vi "__file_name.vi"(8 "comment2":string="m", 9 "種類":u16(ring)=12 items=["LOopt", "LO sweep", "I-V", "I-V NOLO", "I-V Trx", "SP", "YIG", "SBR", "allan", "Gain comp", "Cross Talk", "-----", "A_YIG", "A_SBR", "AL_allan", "AL_fft", "AL_temp", "AL_data", "shapiro", "JC", "htr", "A_SP"], 10 "Control":T2={"GPIB_ATT"="28", "6501Dev#"=1, "GPIB_SP"="18", "GPIB_PM"="13", "GPIB_DSA"="11", "GPIB_DMM (TPD)"="23", "GPIB_MPI"="COM5", "mortor設定"=[{"Axis"=0, "ID"=0, "HIspeed"=200.0, "LOspeed"=100.0, "ACCEL(ms)"=100.0, "Sratio"=50.0, "フリーラン\n"=FALSE, "文字列"="DSB HOT/COLD"}, {"Axis"=1, "ID"=0, "HIspeed"=4.0, "LOspeed"=4.0, "ACCEL(ms)"=100.0, "Sratio"=50.0, "フリーラン\n"=TRUE, "文字列"="SubMM Att"}, {"Axis"=0, "ID"=0, "HIspeed"=200.0, "LOspeed"=100.0, "ACCEL(ms)"=100.0, "Sratio"=50.0, "フリーラン\n"=FALSE, "文字列"="MPI Port1"}, {"Axis"=1, "ID"=0, "HIspeed"=200.0, "LOspeed"=100.0, "ACCEL(ms)"=100.0, "Sratio"=50.0, "フリーラン\n"=FALSE, "文字列"="MPI Port2"}, {"Axis"=1, "ID"=0, "HIspeed"=200.0, "LOspeed"=100.0, "ACCEL(ms)"=100.0, "Sratio"=50.0, "フリーラン\n"=TRUE, "文字列"="gainComp"}], "DATAパス"=path "L:/cartridge/assembly/SN03/03-13/110628_WCADSB_P0", "DBパス "=path "Z:/band10/Labview_ALMA/MIX95/test", "comment"="110628_WCADSB_P0", "ColdCarts"="003601", "Th"=299.0, "Tc"=83.0, "Set_SIS_volt"=2.1, "Offset"=0.0, "control"=0, "FreqLO"=799.0, "Set_Mag_Cur"=8.86861313868613, "MPI offset(mm)"=23.166, "HOT/COLD"=0} {"HOT/COLD" items=["DSB", "SBR (Cart.)", "GainComp", "SBR (MIX)"]; "control" items=["CLOSE LOOP", "OPEN LOOP", "Not Control"]}, 11 "Bias_LO_equip":T1={"Node address"=19, "CAN Interface"="CAN0", "Cartridge band"=10, "Slave Node in"={"Address"=19, "Serial Number"=[16, -88, -112, 75, 1, 8, 0, 24]}, "ObjHandle out"=93257792, "POL"=0, "sb"=1, "GPIB_SM (SIS S,V)"="24", "GPIB_DMM (SIS I)"="22", "GPIB_SM (MAG I) "="25", "GPIB_SG(LO)"="19", "GPIB_PW (PAMP) "="6", "GPIB_TMP1(8ch)"="12", "GPIB_TMP2(2ch)  "="13", "WCA_avg"=10, "Rsen"=10.0, "BiasModule"=1, "LOModule "=2, "WCA_LO_FREQ_SET"={"YTO Low freq. [GHz]"=14.66, "YTO High freq. [GHz]"=17.5, "Kvco"=1, "Lock Pol."=0, "SET LO FREQ"=97.111115, "Multiplier"=6.0, "YTO (HEX)"=2196, "YTO ( FREQ)"=16.18299, "NULL PLL INTEGRATOR"=FALSE}, "Res for"=0} {"Res for" items=["none", "series res", "parallel res"]; "WCA_LO_FREQ_SET"."YTO ( FREQ)" min=25 max=150 step=0.0001 format="%.3f"; "WCA_LO_FREQ_SET"."Multiplier" min=3 max=6 step=3; "WCA_LO_FREQ_SET"."SET LO FREQ" min=25 max=150 step=0.0001 format="%.3f"; "WCA_LO_FREQ_SET"."Lock Pol." items=["Lower", "Upper"]; "WCA_LO_FREQ_SET"."Kvco" items=["7.5MHz/V", "15MHz/V"]; "WCA_LO_FREQ_SET"."YTO High freq. [GHz]" format="%.3f"; "WCA_LO_FREQ_SET"."YTO Low freq. [GHz]" format="%.3f"; "LOModule" items=["Manual Gunn+PAMP"=0, "PLL GUNN+PAMP"=5, "B10Lab LO"=1, "WCA LO"=2, ""=3, "YIG発信器"=4, "none"=99]; "BiasModule" items=["B10Lab Bias"=0, "WCA BiasModule"=1, "none"=99]; "Slave Node in"."Serial Number" format="%.0x"; "Slave Node in"."Address" format="%.0x"; "Cartridge band" max=10 step=1; "Node address" format="%.0x"}) -> (3 "file_name":string="YIG_799.00_120_110628_WCADSB_P0m.csv")   [LabVIEW 2017]
panel:
  # "LO freq. [GHz]"
  # "YTO LOW\n/High Freq."
  # "ZERO Intgrtr"
  # "Node Address"
  # "Serial Number"
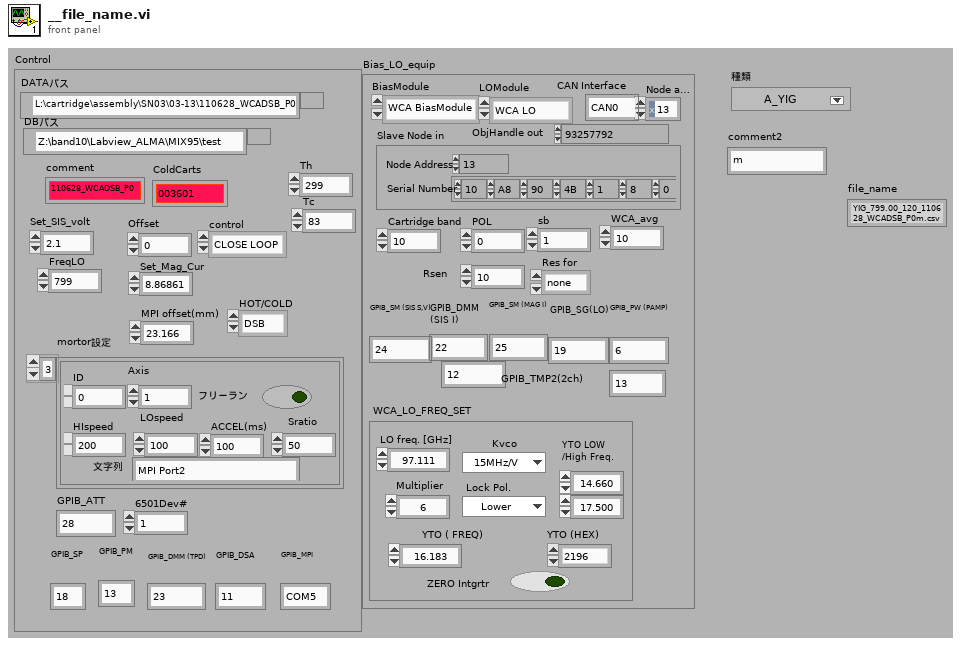
[diagram p1: front panel]
types:
  T1 = cluster{"Node address":u16, "CAN Interface":string, "Cartridge band":u32, "Slave Node in":cluster{"Address":i16, "Serial Number":i8[]}, "ObjHandle out":u32, "POL":u32, "sb":u32, "GPIB_SM (SIS S,V)":string, "GPIB_DMM (SIS I)":string, "GPIB_SM (MAG I) ":string, "GPIB_SG(LO)":string, "GPIB_PW (PAMP) ":string, "GPIB_TMP1(8ch)":string, "GPIB_TMP2(2ch)  ":string, "WCA_avg":i32, "Rsen":dbl, "BiasModule":u16, "LOModule ":u16, "WCA_LO_FREQ_SET":cluster{"YTO Low freq. [GHz]":sgl, "YTO High freq. [GHz]":sgl, "Kvco":u16, "Lock Pol.":u16, "SET LO FREQ":sgl, "Multiplier":sgl, "YTO (HEX)":u16, "YTO ( FREQ)":sgl, "NULL PLL INTEGRATOR":bool}, "Res for":u16}
  T2 = cluster{"GPIB_ATT":string, "6501Dev#":i16, "GPIB_SP":string, "GPIB_PM":string, "GPIB_DSA":string, "GPIB_DMM (TPD)":string, "GPIB_MPI":string, "mortor設定":cluster{"Axis":i16, "ID":i16, "HIspeed":dbl, "LOspeed":dbl, "ACCEL(ms)":dbl, "Sratio":dbl, "フリーラン\n":bool, "文字列":string}[], "DATAパス":path, "DBパス ":path, "comment":string, "ColdCarts":string, "Th":dbl, "Tc":dbl, "Set_SIS_volt":dbl, "Offset":dbl, "control":u16, "FreqLO":dbl, "Set_Mag_Cur":dbl, "MPI offset(mm)":dbl, "HOT/COLD":u16}
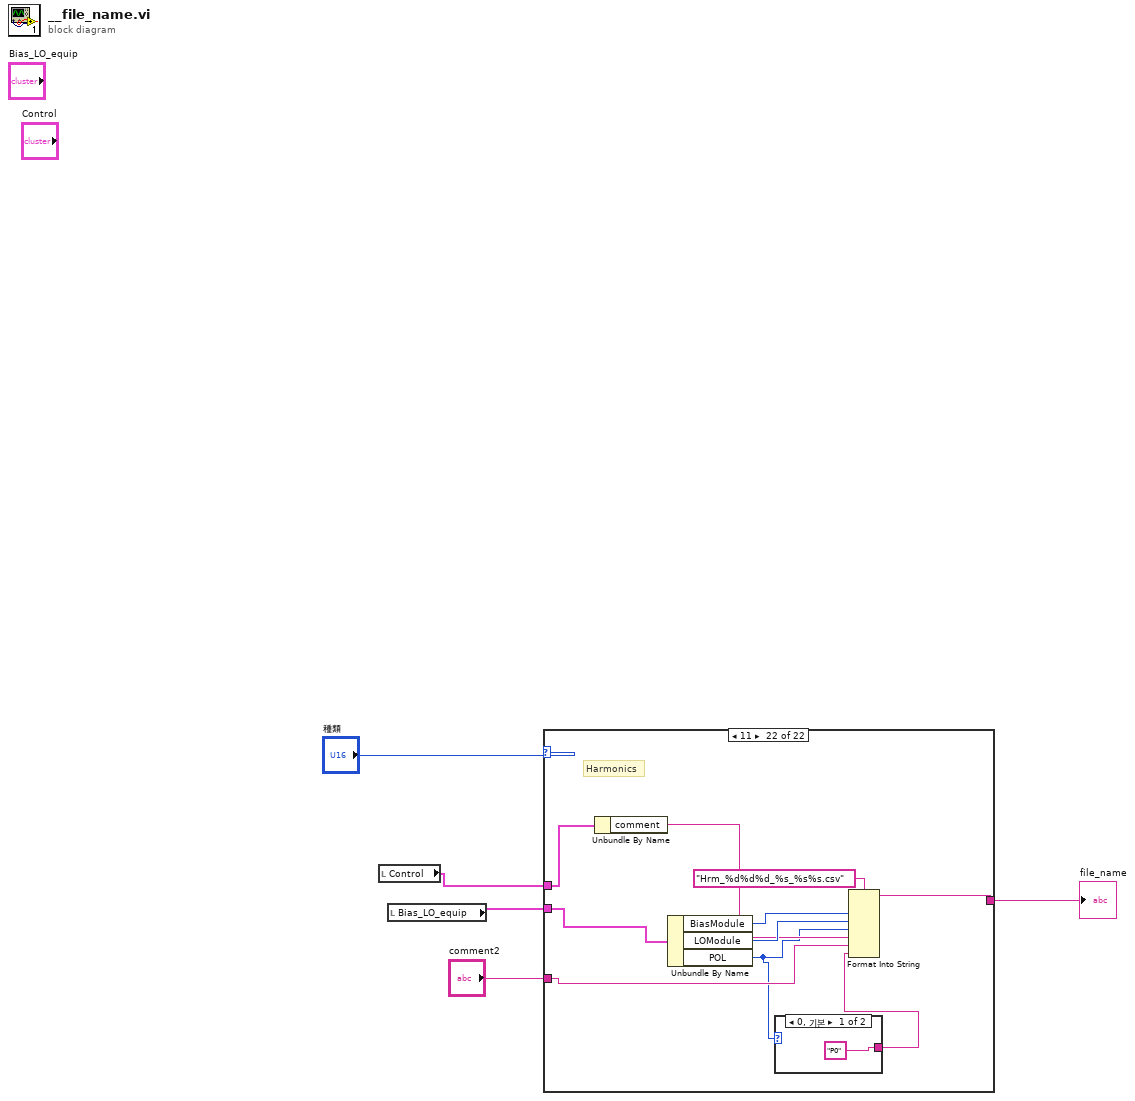
[diagram p0: block diagram]
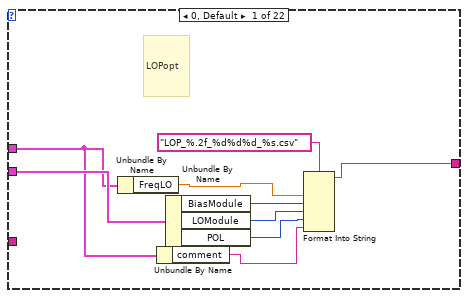
[diagram p2: hidden frame]
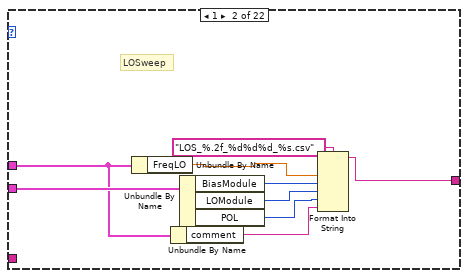
[diagram p3: hidden frame]
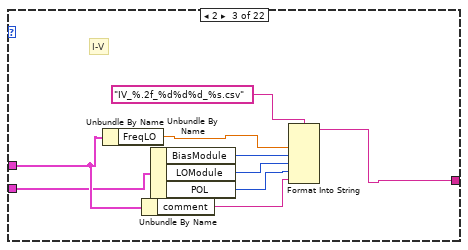
[diagram p4: hidden frame]
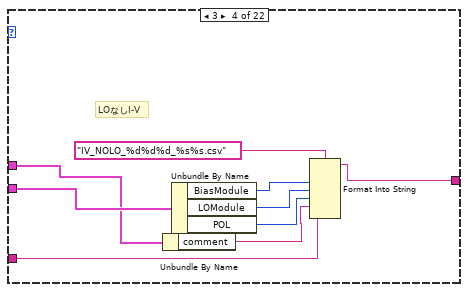
[diagram p5: hidden frame]
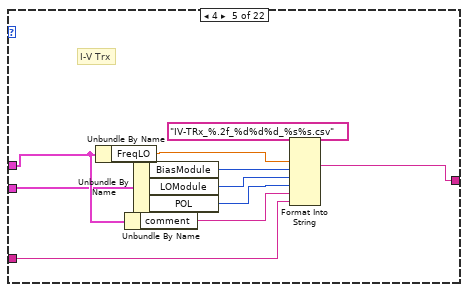
[diagram p6: hidden frame]
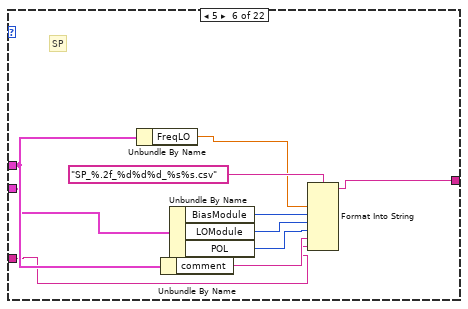
[diagram p7: hidden frame]
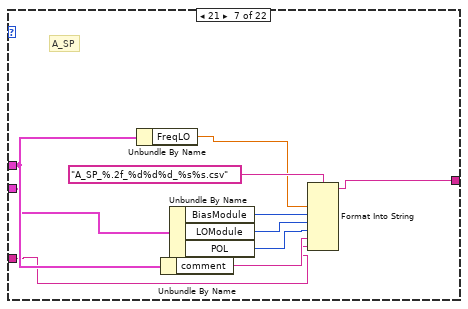
[diagram p8: hidden frame]
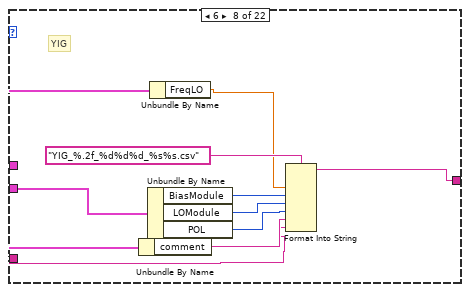
[diagram p9: hidden frame]
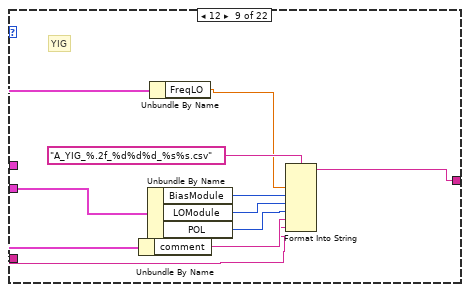
[diagram p10: hidden frame]
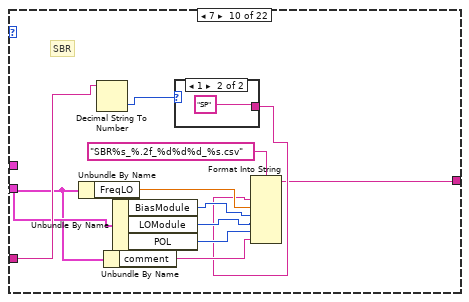
[diagram p11: hidden frame]
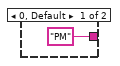
[diagram p12: hidden frame]
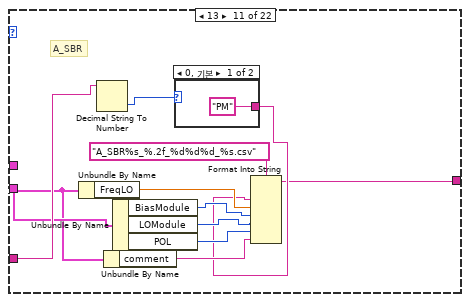
[diagram p13: hidden frame]
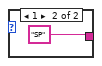
[diagram p14: hidden frame]
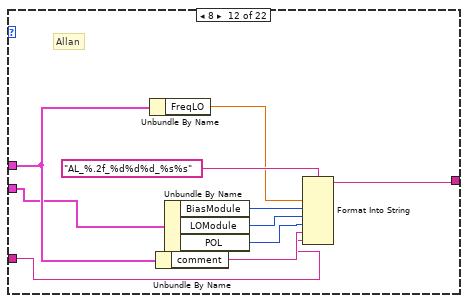
[diagram p15: hidden frame]
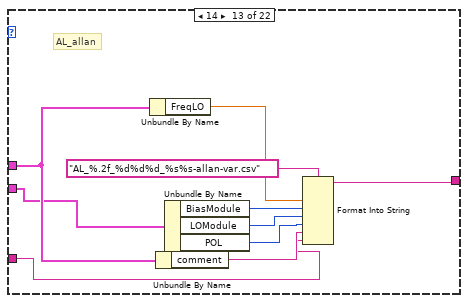
[diagram p16: hidden frame]
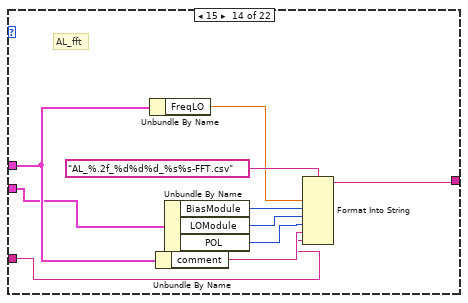
[diagram p17: hidden frame]
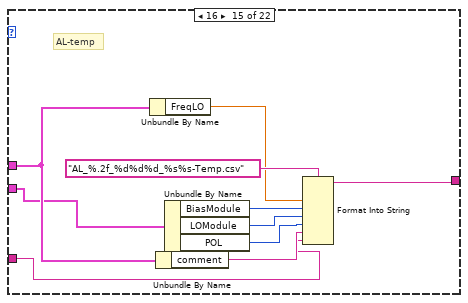
[diagram p18: hidden frame]
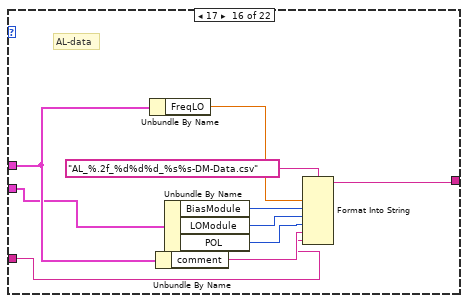
[diagram p19: hidden frame]
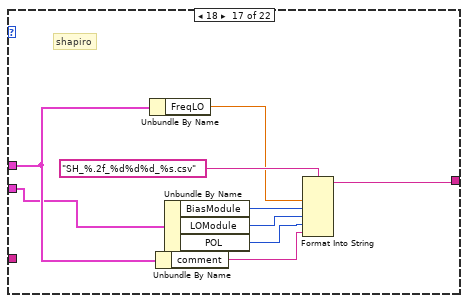
[diagram p20: hidden frame]
diagram:
  n1 = local read "Control"() -> (w4:T2)
  n2 = local read "Bias_LO_equip"() -> (w5:T1)
  n3 = case shown="11" "種類" {
    tunnel: w5 -> [w9 w22 w26 w36 w44 w54 w64 w74 w84 w94 w108 w122 w132 w142 w152 w162 w171 w181 w188 w197 w206 w220]
    tunnel: w4 -> [w7 w16 w27 w35 w45 w55 w65 w75 w85 w93 w107 w123 w133 w143 w153 w163 w172 w182 w189 w198 w207 w218]
    tunnel: [w8 w17 w25 w33 w43 w53 w63 w72 w82 w92 w106 w120 w130 w140 w150 w160 w170 w180 w187 w195 w205 w219] -> w2
    tunnel: "comment2" -> [_ _ _ w34 w42 w52 w62 w73 w83 w97 w111 w121 w131 w141 w151 w161 _ _ _ w196 _ w216]
    frame 0, Default {
      # "LOPopt"
      n4 = Unbundle By Name(w7) -> ("FreqLO"=w10:dbl)
      n5 = Unbundle By Name(w7) -> ("comment"=w6:string)
      n6 = Unbundle By Name(w9) -> ("BiasModule"=w13:u16, "LOModule"=w12:u16, "POL"=w11:u32)
      n7 = Format Into String(format string="LOP_%.2f_%d%d%d_%s.csv", w10, w13, w12, w11, w6) -> (resulting string=w8:string)  [unwired: 2 in, 1 out]
    }
    frame 1 {
      # "LOSweep"
      n8 = Unbundle By Name(w16) -> ("FreqLO"=w18:dbl)
      n9 = Unbundle By Name(w16) -> ("comment"=w15:string)
      n10 = Unbundle By Name(w22) -> ("BiasModule"=w21:u16, "LOModule"=w20:u16, "POL"=w19:u32)
      n11 = Format Into String(format string="LOS_%.2f_%d%d%d_%s.csv", w18, w21, w20, w19, w15) -> (resulting string=w17:string)  [unwired: 2 in, 1 out]
    }
    frame 2 {
      # "I-V"
      n12 = Unbundle By Name(w27) -> ("FreqLO"=w28:dbl)
      n13 = Unbundle By Name(w27) -> ("comment"=w29:string)
      n14 = Unbundle By Name(w26) -> ("BiasModule"=w32:u16, "LOModule"=w31:u16, "POL"=w30:u32)
      n15 = Format Into String(format string="IV_%.2f_%d%d%d_%s.csv", w28, w32, w31, w30, w29) -> (resulting string=w25:string)  [unwired: 2 in, 1 out]
    }
    frame 3 {
      # "LOなしI-V"
      n16 = Unbundle By Name(w35) -> ("comment"=w38:string)
      n17 = Unbundle By Name(w36) -> ("BiasModule"=w41:u16, "LOModule"=w40:u16, "POL"=w39:u32)
      n18 = Format Into String(format string="IV_NOLO_%d%d%d_%s%s.csv", w41, w40, w39, w38, w34) -> (resulting string=w33:string)  [unwired: 2 in, 1 out]
    }
    frame 4 {
      # "I-V Trx"
      n19 = Unbundle By Name(w45) -> ("FreqLO"=w46:dbl)
      n20 = Unbundle By Name(w45) -> ("comment"=w47:string)
      n21 = Unbundle By Name(w44) -> ("BiasModule"=w50:u16, "LOModule"=w49:u16, "POL"=w48:u32)
      n22 = Format Into String(format string="IV-TRx_%.2f_%d%d%d_%s%s.csv", w46, w50, w49, w48, w47, w42) -> (resulting string=w43:string)  [unwired: 2 in, 1 out]
    }
    frame 5 {
      # "SP"
      n23 = Unbundle By Name(w55) -> ("FreqLO"=w56:dbl)
      n24 = Unbundle By Name(w55) -> ("comment"=w57:string)
      n25 = Unbundle By Name(w54) -> ("BiasModule"=w60:u16, "LOModule"=w59:u16, "POL"=w58:u32)
      n26 = Format Into String(format string="SP_%.2f_%d%d%d_%s%s.csv", w56, w60, w59, w58, w57, w52) -> (resulting string=w53:string)  [unwired: 2 in, 1 out]
    }
    frame 21 {
      # "A_SP"
      n27 = Unbundle By Name(w65) -> ("FreqLO"=w66:dbl)
      n28 = Unbundle By Name(w65) -> ("comment"=w67:string)
      n29 = Unbundle By Name(w64) -> ("BiasModule"=w70:u16, "LOModule"=w69:u16, "POL"=w68:u32)
      n30 = Format Into String(format string="A_SP_%.2f_%d%d%d_%s%s.csv", w66, w70, w69, w68, w67, w62) -> (resulting string=w63:string)  [unwired: 2 in, 1 out]
    }
    frame 6 {
      # "YIG"
      n31 = Unbundle By Name(w75) -> ("comment"=w77:string)
      n32 = Unbundle By Name(w74) -> ("BiasModule"=w80:u16, "LOModule"=w79:u16, "POL"=w78:u32)
      n33 = Unbundle By Name(w75) -> ("FreqLO"=w76:dbl)
      n34 = Format Into String(format string="YIG_%.2f_%d%d%d_%s%s.csv", w76, w80, w79, w78, w77, w73) -> (resulting string=w72:string)  [unwired: 2 in, 1 out]
    }
    frame 12 {
      # "YIG"
      n35 = Unbundle By Name(w85) -> ("comment"=w87:string)
      n36 = Unbundle By Name(w84) -> ("BiasModule"=w90:u16, "LOModule"=w89:u16, "POL"=w88:u32)
      n37 = Unbundle By Name(w85) -> ("FreqLO"=w86:dbl)
      n38 = Format Into String(format string="A_YIG_%.2f_%d%d%d_%s%s.csv", w86, w90, w89, w88, w87, w83) -> (resulting string=w82:string)  [unwired: 2 in, 1 out]
    }
    frame 7 {
      # "SBR"
      n39 = Unbundle By Name(w93) -> ("FreqLO"=w98:dbl)
      n40 = Decimal String To Number(string=w97) -> (number=w96:i32)  [unwired: 2 in, 1 out]
      n41 = Unbundle By Name(w93) -> ("comment"=w102:string)
      n42 = Unbundle By Name(w94) -> ("BiasModule"=w101:u16, "LOModule"=w100:u16, "POL"=w99:u32)
      n43 = case shown="1" w96 {
        tunnel: ["PM" "SP"] -> w95
        frame 0, Default {
        }
        frame 1 {
        }
      }
      n44 = Format Into String(format string="SBR%s_%.2f_%d%d%d_%s.csv", w95, w98, w101, w100, w99, w102) -> (resulting string=w92:string)  [unwired: 2 in, 1 out]
    }
    frame 13 {
      # "A_SBR"
      n45 = Unbundle By Name(w107) -> ("FreqLO"=w112:dbl)
      n46 = Decimal String To Number(string=w111) -> (number=w110:i32)  [unwired: 2 in, 1 out]
      n47 = Unbundle By Name(w107) -> ("comment"=w116:string)
      n48 = Unbundle By Name(w108) -> ("BiasModule"=w115:u16, "LOModule"=w114:u16, "POL"=w113:u32)
      n49 = case shown="0, 기본" w110 {
        tunnel: ["PM" "SP"] -> w109
        frame 0, Default {
        }
        frame 1 {
        }
      }
      n50 = Format Into String(format string="A_SBR%s_%.2f_%d%d%d_%s.csv", w109, w112, w115, w114, w113, w116) -> (resulting string=w106:string)  [unwired: 2 in, 1 out]
    }
    frame 8 {
      # "Allan"
      n51 = Unbundle By Name(w123) -> ("FreqLO"=w124:dbl)
      n52 = Unbundle By Name(w123) -> ("comment"=w125:string)
      n53 = Unbundle By Name(w122) -> ("BiasModule"=w128:u16, "LOModule"=w127:u16, "POL"=w126:u32)
      n54 = Format Into String(format string="AL_%.2f_%d%d%d_%s%s", w124, w128, w127, w126, w125, w121) -> (resulting string=w120:string)  [unwired: 2 in, 1 out]
    }
    frame 14 {
      # "AL_allan"
      n55 = Unbundle By Name(w133) -> ("FreqLO"=w134:dbl)
      n56 = Unbundle By Name(w133) -> ("comment"=w135:string)
      n57 = Unbundle By Name(w132) -> ("BiasModule"=w138:u16, "LOModule"=w137:u16, "POL"=w136:u32)
      n58 = Format Into String(format string="AL_%.2f_%d%d%d_%s%s-allan-var.csv", w134, w138, w137, w136, w135, w131) -> (resulting string=w130:string)  [unwired: 2 in, 1 out]
    }
    frame 15 {
      # "AL_fft"
      n59 = Unbundle By Name(w143) -> ("FreqLO"=w144:dbl)
      n60 = Unbundle By Name(w143) -> ("comment"=w145:string)
      n61 = Unbundle By Name(w142) -> ("BiasModule"=w148:u16, "LOModule"=w147:u16, "POL"=w146:u32)
      n62 = Format Into String(format string="AL_%.2f_%d%d%d_%s%s-FFT.csv", w144, w148, w147, w146, w145, w141) -> (resulting string=w140:string)  [unwired: 2 in, 1 out]
    }
    frame 16 {
      # "AL-temp"
      n63 = Unbundle By Name(w153) -> ("FreqLO"=w154:dbl)
      n64 = Unbundle By Name(w153) -> ("comment"=w155:string)
      n65 = Unbundle By Name(w152) -> ("BiasModule"=w158:u16, "LOModule"=w157:u16, "POL"=w156:u32)
      n66 = Format Into String(format string="AL_%.2f_%d%d%d_%s%s-Temp.csv", w154, w158, w157, w156, w155, w151) -> (resulting string=w150:string)  [unwired: 2 in, 1 out]
    }
    frame 17 {
      # "AL-data"
      n67 = Unbundle By Name(w163) -> ("FreqLO"=w164:dbl)
      n68 = Unbundle By Name(w163) -> ("comment"=w165:string)
      n69 = Unbundle By Name(w162) -> ("BiasModule"=w168:u16, "LOModule"=w167:u16, "POL"=w166:u32)
      n70 = Format Into String(format string="AL_%.2f_%d%d%d_%s%s-DM-Data.csv", w164, w168, w167, w166, w165, w161) -> (resulting string=w160:string)  [unwired: 2 in, 1 out]
    }
    frame 18 {
      # "shapiro"
      n71 = Unbundle By Name(w172) -> ("FreqLO"=w173:dbl)
      n72 = Unbundle By Name(w172) -> ("comment"=w174:string)
      n73 = Unbundle By Name(w171) -> ("BiasModule"=w177:u16, "LOModule"=w176:u16, "POL"=w175:u32)
      n74 = Format Into String(format string="SH_%.2f_%d%d%d_%s.csv", w173, w177, w176, w175, w174) -> (resulting string=w170:string)  [unwired: 2 in, 1 out]
    }
    frame 19 {
      # "JC"
      n75 = Unbundle By Name(w182) -> ("comment"=w183:string)
      n76 = Unbundle By Name(w181) -> ("BiasModule"=w185:u16, "LOModule"=w184:u16, "POL"=w179:u32)
      n77 = Format Into String(format string="JC_%d%d%d_%s.csv", w185, w184, w179, w183) -> (resulting string=w180:string)  [unwired: 2 in, 1 out]
    }
    frame 20 {
      # "Defluxhtr"
      n78 = Unbundle By Name(w189) -> ()  [unwired: 1 out]
      n79 = Unbundle By Name(w189) -> ("comment"=w190:string)
      n80 = Unbundle By Name(w188) -> ("BiasModule"=w193:u16, "LOModule"=w192:u16, "POL"=w191:u32)
      n81 = Format Into String(format string="HTR_%d%d%d_%s.csv", w193, w192, w191, w190) -> (resulting string=w187:string)  [unwired: 2 in, 1 out]
    }
    frame 9 {
      # "GainComp"
      n82 = Unbundle By Name(w198) -> ("FreqLO"=w199:dbl)
      n83 = Unbundle By Name(w198) -> ("comment"=w200:string)
      n84 = Unbundle By Name(w197) -> ("BiasModule"=w203:u16, "LOModule"=w202:u16, "POL"=w201:u32)
      n85 = Format Into String(format string="GC_%.2f_%d%d%d_%s%s.csv", w199, w203, w202, w201, w200, w196) -> (resulting string=w195:string)  [unwired: 2 in, 1 out]
    }
    frame 10 {
      # "Crosstalk"
      n86 = Unbundle By Name(w207) -> ("FreqLO"=w208:dbl)
      n87 = Unbundle By Name(w207) -> ("comment"=w209:string)
      n88 = Unbundle By Name(w206) -> ("BiasModule"=w212:u16, "LOModule"=w211:u16, "POL"=w210:u32)
      n89 = Format Into String(format string="xtk_%.2f_%d%d%d_%s.csv", w208, w212, w211, w210, w209) -> (resulting string=w205:string)  [unwired: 2 in, 1 out]
    }
    frame 11 {
      # "Harmonics"
      n90 = Unbundle By Name(w218) -> ("comment"=w217:string)
      n91 = Unbundle By Name(w220) -> ("BiasModule"=w222:u16, "LOModule"=w221:u16, "POL"=w215:u32)
      n92 = case shown="0, 기본" w215 {
        tunnel: ["P0" "P1"] -> w214
        frame 0, Default {
        }
        frame 1 {
        }
      }
      n93 = Format Into String(format string="Hrm_%d%d%d_%s_%s%s.csv", w222, w221, w215, w217, w216, w214) -> (resulting string=w219:string)  [unwired: 2 in, 1 out]
    }
  }
  "file_name" <- w2
